vi "oa_SCL Autoscale XY.vi"(1 "axis attributes":T1={"x minimum"=0.0, "x maximum"=0.0, "x log?"=FALSE, "x precision"=1, "x format"=enum."Decimal", "y minimum"=0.0, "y maximum"=0.0, "y log?"=FALSE, "y precision"=1, "y format"=enum."Decimal"} {"x minimum" format="%0.2f"; "x maximum" format="%0.2f"; "y minimum" format="%0.2f"; "y maximum" format="%0.2f"}, 2 "xy data":cluster{"x":dbl, "y":dbl}[](array[cluster]) {"y" format="%0.2f"; "x" format="%0.2f"}) -> (0 "axis attributes":T1={"x minimum"=0.0, "x maximum"=0.0, "x log?"=FALSE, "x precision"=1, "x format"=enum."Decimal", "y minimum"=0.0, "y maximum"=0.0, "y log?"=FALSE, "y precision"=1, "y format"=enum."Decimal"} {"x minimum" format="%0.2f"; "x maximum" format="%0.2f"; "y minimum" format="%0.2f"; "y maximum" format="%0.2f"})   [LabVIEW 2017]
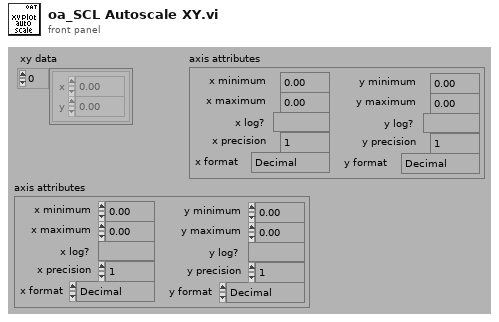
[diagram p1: front panel]
types:
  T1 = cluster{"x minimum":dbl, "x maximum":dbl, "x log?":bool, "x precision":u8, "x format":enum8{"Decimal", "Scientific", "Engineering", "Binary", "Octal", "Hex"}, "y minimum":dbl, "y maximum":dbl, "y log?":bool, "y precision":u8, "y format":enum8{"Decimal", "Scientific", "Engineering", "Binary", "Octal", "Hex"}}
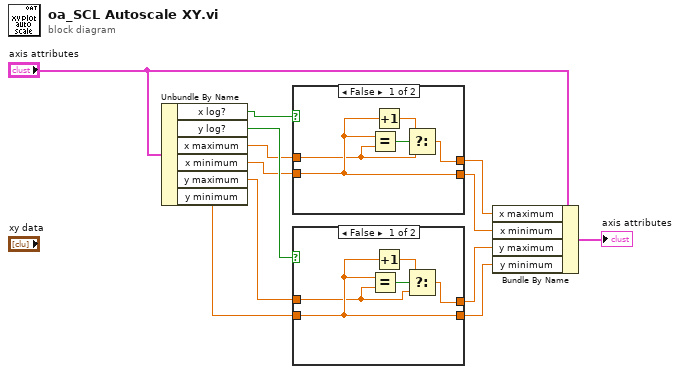
[diagram p0: block diagram]
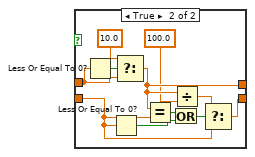
[diagram p2: hidden frame]
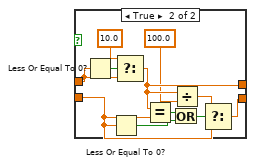
[diagram p3: hidden frame]
diagram:
  n1 = Unbundle By Name("axis attributes") -> ("x log?"=w10:bool, "y log?"=w7:bool, "x maximum"=w4:dbl, "x minimum"=w3:dbl, "y maximum"=w2:dbl, "y minimum"=w1:dbl)
  n2 = case shown="False" w10 {
    tunnel: w4 -> [w13 w26]
    tunnel: w3 -> [w17 w22]
    tunnel: [w17 w21] -> w12
    tunnel: [w14 w20] -> w11
    frame False {
      n3 = Equal?(x=w17, y=w13) -> (x = y?=w16:bool)
      n4 = Increment(x=w17) -> (x+1=w15:dbl)
      n5 = Select(t=w15, s=w16, f=w13) -> (s? t:f=w14:dbl)
    }
    frame True {
      n6 = Less Or Equal To 0?(x=w26) -> (x <= 0?=w27:bool)
      n7 = Less Or Equal To 0?(x=w22) -> (x <= 0?=w25:bool)
      n8 = Select(t=10.0, s=w27, f=w26) -> (s? t:f=w20:dbl)
      n9 = Equal?(x=w20, y=w22) -> (x = y?=w23:bool)
      n10 = Or(x=w23, y=w25) -> (x .or. y?=w24:bool)
      n11 = Divide(x=w20, y=100.0) -> (x/y=w18:dbl)
      n12 = Select(t=w18, s=w24, f=w22) -> (s? t:f=w21:dbl)
    }
  }
  n13 = case shown="False" w7 {
    tunnel: w2 -> [w29 w42]
    tunnel: w1 -> [w33 w38]
    tunnel: [w33 w37] -> w8
    tunnel: [w30 w36] -> w9
    frame False {
      n14 = Equal?(x=w33, y=w29) -> (x = y?=w32:bool)
      n15 = Increment(x=w33) -> (x+1=w31:dbl)
      n16 = Select(t=w31, s=w32, f=w29) -> (s? t:f=w30:dbl)
    }
    frame True {
      n17 = Less Or Equal To 0?(x=w42) -> (x <= 0?=w43:bool)
      n18 = Less Or Equal To 0?(x=w38) -> (x <= 0?=w41:bool)
      n19 = Select(t=10.0, s=w43, f=w42) -> (s? t:f=w36:dbl)
      n20 = Equal?(x=w36, y=w38) -> (x = y?=w39:bool)
      n21 = Or(x=w39, y=w41) -> (x .or. y?=w40:bool)
      n22 = Divide(x=w36, y=100.0) -> (x/y=w34:dbl)
      n23 = Select(t=w34, s=w40, f=w38) -> (s? t:f=w37:dbl)
    }
  }
  n24 = Bundle By Name(cluster="axis attributes", "x maximum"=w11, "x minimum"=w12, "y maximum"=w9, "y minimum"=w8) -> (→"axis attributes":T1)
